vi "DoLayoutChange.vi"(6 "Column":i32, 8 "error in (no error)":errorcluster, 9 "Tbl Refnum":refnum<vi>, 10 "Layout index":i32, 11 "Column in":refnum<class "Column.lvclass">) -> (0 "error out":errorcluster, 2 "Set Width":u32, 3 "Column out":refnum<class "Column.lvclass">)   [LabVIEW 2013, in "Column.lvclass"]
doc: "Set Column width in SetList Table. If \"Layout index\" is non-negative, the user-configured layouts stored in the Column objects are read so that some columns are hidden. For negative \"layout index\" all columns are shown at their specified widths."
uses:
  Column.lvclass
  <vilib>/Utility/miscctls.llb/LVRowAndColumnTypeDef.ctl
  Column.lvclass/Column.ctl
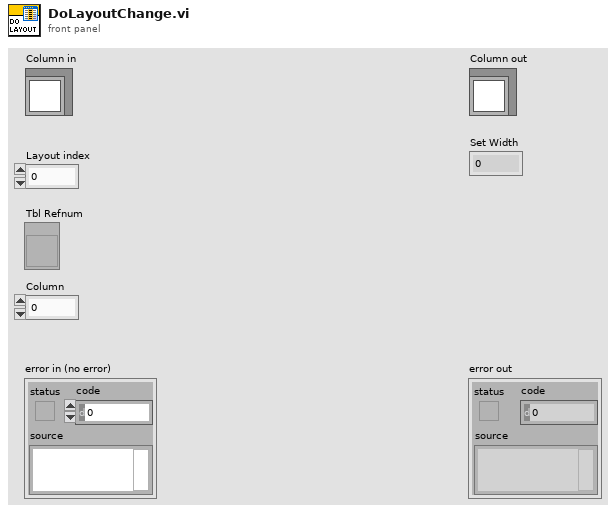
[diagram p1: front panel]
types:
  T1 = typedef "LVRowAndColumnTypeDef.ctl" = cluster{"Row":i32, "Column":i32}
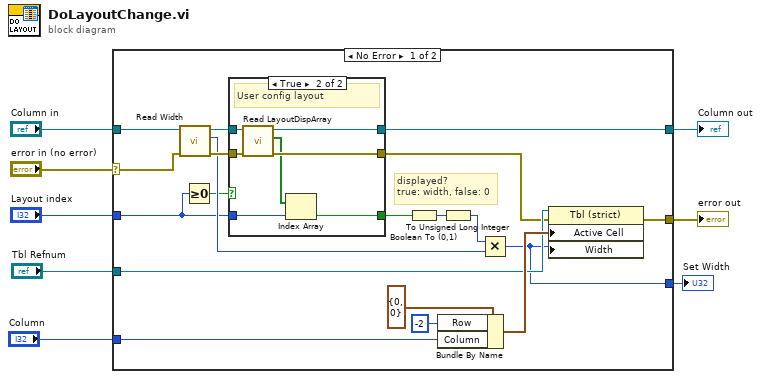
[diagram p0: block diagram]
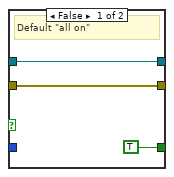
[diagram p2: hidden frame]
diagram:
  n1 = case shown="No Error" "error in (no error)" {
    selector: "error in (no error)" -> [w18 w39]
    tunnel: [w20 w39] -> w7
    tunnel: [w16 w38] -> w5
    tunnel: "Column in" -> [w19 w38]
    tunnel: "Column" -> [w22 _]
    tunnel: "Tbl Refnum" -> [w21 _]
    tunnel: "Layout index" -> [w11 _]
    tunnel: [w9 _] -> w1
    frame No Error {
      # "displayed? \ntrue: width, false: 0"
      n2 = call "Read Width.vi"("error in (no error)"=w18, "Column in"=w19) -> ("error out"=w15:errorcluster, "Width"=w13:u32, "Column out"=w17:refnum<class "Column.lvclass">)  [unwired: 7 in]
      n3 = Greater Or Equal To 0?(x=w11) -> (x >= 0?=w10:bool)
      n4 = case shown="True" w10 {
        tunnel: w17 -> [w30 w37]
        tunnel: [w30 w36] -> w16
        tunnel: w15 -> [w29 w35]
        tunnel: [w29 w34] -> w14
        tunnel: w11 -> [_ w32]
        tunnel: [TRUE w31] -> w12
        frame False {
          # "Default \"all on\""
        }
        frame True {
          # "User config layout"
          n5 = call "Read LayoutDispArray.vi"("error in (no error)"=w35, "Column in"=w37) -> ("error out"=w34:errorcluster, "Layout disp? array"=w33:bool[], "Column out"=w36:refnum<class "Column.lvclass">)  [unwired: 7 in]
          n6 = Index Array(array=w33, index=w32) -> (element=w31:bool)
        }
      }
      n7 = Boolean To (0,1)(Boolean=w12) -> (0, 1=w24:i16)
      n8 = Bundle By Name(cluster=T1 {"Row"=0, "Column"=0} ("Active Cell:Active Cell"), "Row"=-2, "Column"=w22) -> (w25:T1)
      n9 = To Unsigned Long Integer(number=w24) -> (unsigned 32bit integer=w23:u32)
      n10 = Multiply(x=w23, y=w13) -> (x*y=w9:u32)
      n11 = property on="Property Node" class="Tbl (strict)"(reference=w21, error in=w14, "Active Cell"=w25, "Width"=w9) -> (error out=w20:errorcluster)  [unwired: 1 out]
    }
    frame Error {
    }
  }
  "error out" <- w7
  "Column out" <- w5
  "Set Width" <- w1
